vi "Get Object by Name.vi"(8 "error in":errorcluster, 10 "Name":string, 11 "Button Manager in":refnum<class "Button Manager.lvclass">) -> (0 "error out":errorcluster, 1 "Ctl Ref":refnum<vi>, 2 "Button Object":T1, 3 "Button Manager out":refnum<class "Button Manager.lvclass">)   [LabVIEW 2022 SP3, in "Navigation.lvlib" / "Button Manager.lvclass"]
doc: "____\nHAMPEL SOFTWARE ENGINEERING v2.6.0 (2023-12-19 10:54)"
uses:
  Button Manager.lvclass
  Top Control.ctl
  Sub Control.ctl
  Button Manager.lvclass/Button Manager.ctl
  Button Def.ctl
  <vilib>/Utility/error.llb/Error Cluster From Error Code.vi
  <vilib>/ErrorRing/Error Ring.xnode
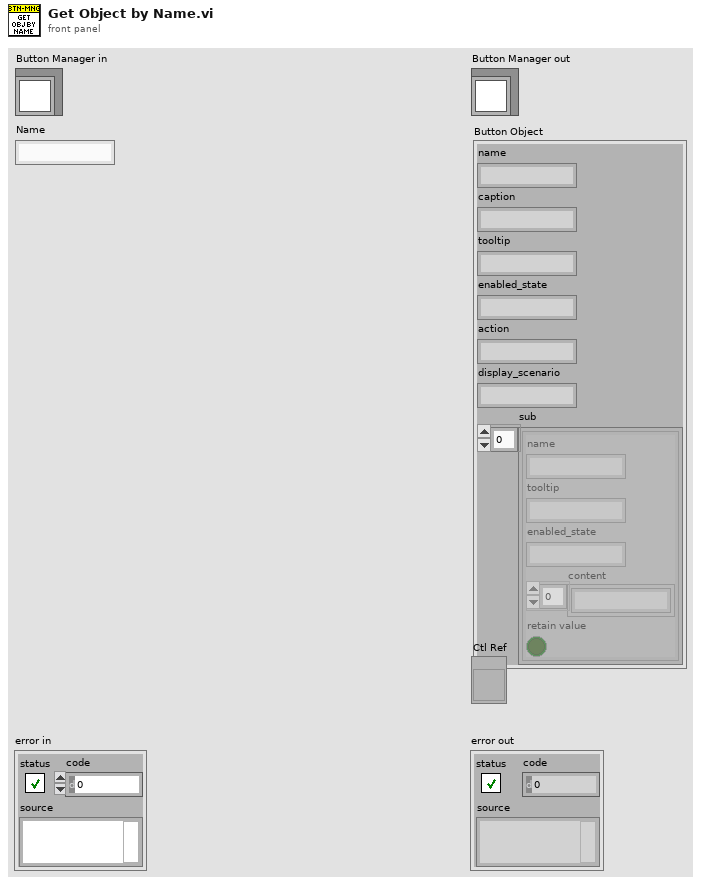
[diagram p1: front panel]
types:
  T1 = typedef "Navigation.lvlib/Button Manager.lvclass/Top Control.ctl" = cluster{"name":string, "caption":string, "tooltip":string, "enabled_state":string, "action":string, "display_scenario":string, "sub":T2[]}
  T2 = typedef "Navigation.lvlib/Button Manager.lvclass/Sub Control.ctl" = cluster{"name":string, "tooltip":string, "enabled_state":string, "content":string[], "retain value":bool}
  T3 = typedef "Navigation.lvlib/Button Manager.lvclass/Button Def.ctl" = cluster{"Top-Ctl Ref":refnum<vi>, "Sub-Ctl Ref":refnum<vi>, "Button Object":T1}
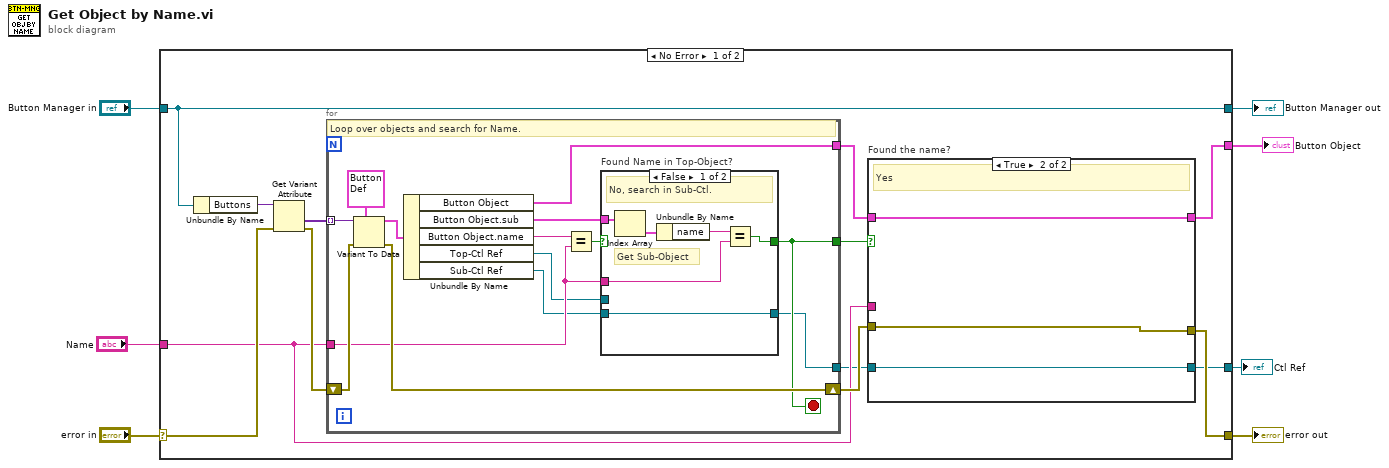
[diagram p0: block diagram]
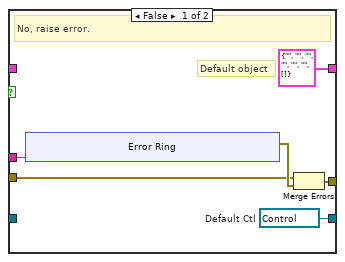
[diagram p2: hidden frame]
diagram:
  n1 = case shown="No Error" "error in" {
    selector: "error in" -> [w17 w60]
    tunnel: [w12 w60] -> w6
    tunnel: [w19 w59] -> w4
    tunnel: "Button Manager in" -> [w19 w59]
    tunnel: "Name" -> [w14 _]
    tunnel: [w10 _] -> w2
    tunnel: [w8 _] -> w1
    frame No Error {
      n2 = Unbundle By Name(w19) -> ("Buttons"=w18:variant)
      n3 = Get Variant Attribute(Variant=w18, error in=w17) -> (values=w16:variant[], error out=w15:errorcluster)  [unwired: 2 in, 2 out]
      n4 = for {
        tunnel: w16 -> [w49] mode=indexing
        tunnel: w14 -> [w44]
        tunnel: [w43] -> w13
        shift-right: [w50] -> w20
        shift-left: w15 -> [w48]
        tunnel: [w40] -> w11
        tunnel: [w37] -> w9
        stop <- w43 stop-if-true
        # "Loop over objects and search for Name."
        n5 = Variant To Data(error in=w48, type=T3 {"Top-Ctl Ref"=refnum, "Sub-Ctl Ref"=refnum, "Button Object"={"name"="", "caption"="", "tooltip"="", "enabled_state"="", "action"="", "display_scenario"="", "sub"=[]}} ("Button Def"), Variant=w49) -> (data=w42:T3, error out=w50:errorcluster)
        n6 = Unbundle By Name(w42) -> ("Button Object"=w40:T1, "Button Object.sub"=w41:T2[], "Button Object.name"=w46:string, "Top-Ctl Ref"=w39:refnum<vi>, "Sub-Ctl Ref"=w38:refnum<vi>)
        n7 = Equal?(x=w46, y=w44) -> (x = y?=w45:bool)
        n8 = case "Found Name in Top-Object?" shown="False" w45 {
          selector: w45 -> [_ w58]
          tunnel: w41 -> [w55 _]
          tunnel: w44 -> [w53 _]
          tunnel: [w52 w58] -> w43
          tunnel: w39 -> [_ w57]
          tunnel: w38 -> [w51 _]
          tunnel: [w51 w57] -> w37
          frame False {
            # "Get Sub-Object"
            # "No, search in Sub-Ctl."
            n9 = Index Array(array=w55) -> (element=w56:T2)  [unwired: 1 in]
            n10 = Unbundle By Name(w56) -> ("name"=w54:string)
            n11 = Equal?(x=w54, y=w53) -> (x = y?=w52:bool)
          }
          frame True {
            # "Yes, don't search in Sub-Ctl."
          }
        }
      }
      n12 = case "Found the name?" shown="True" w13 {
        tunnel: w14 -> [w26 _]
        tunnel: w20 -> [w24 w36]
        tunnel: [w23 w36] -> w12
        tunnel: w11 -> [_ w35]
        tunnel: [T1 {"name"="", "caption"="", "tooltip"="", "enabled_state"="", "action"="", "display_scenario"="", "sub"=[]} ("Button Object") w35] -> w10
        tunnel: [w21 w34] -> w8
        tunnel: w9 -> [_ w34]
        frame False {
          w21 = refnum<vi> refnum  # Default Ctl
          # "Default object"
          # "No, raise error."
          n13 = xnode "Error Ring"("parameter 0"=w26) -> ("error out"=w25:errorcluster)
          n14 = Merge Errors(w24, w25) -> (w23:errorcluster)
        }
        frame True {
          # "Yes"
        }
      }
    }
    frame Error {
    }
  }
  "error out" <- w6
  "Button Manager out" <- w4
  "Button Object" <- w2
  "Ctl Ref" <- w1
